vi "Launcher.vi"() -> ()   [LabVIEW 2024]
uses:
  Support/Traversal Type.ctl
  Tree_class/Tree.lvclass
  Iterator_interface/Iterator.lvclass
  <vilib>/Utility/miscctls.llb/LVRectTypeDef.ctl
  Node_class/Node.lvclass
panel:
  out "TreeSaved":bool
  in  "GoNext":bool
  in  "Save":bool
  in  "Add":bool
  in  "Value":dbl
  in  "TraversalType":T1
  out "TreeElements":dbl[](array[numeric])
  # "TREE VALUES"
  # "Made by Ramazan Burak Korkmaz"
  # "Value"
  # "Traversal\nType"
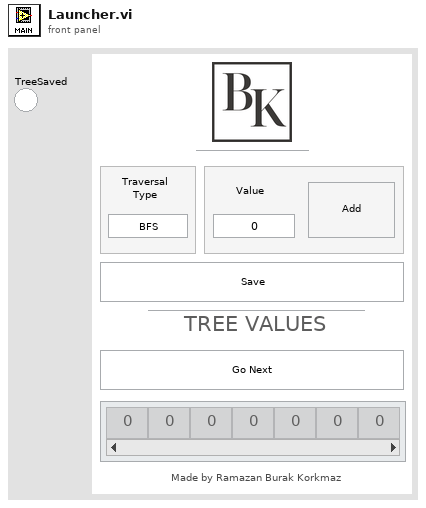
[diagram p1: front panel]
types:
  T1 = typedef "Traversal Type.ctl" = enum16{"BFS", "DFS"}
  T2 = enum8{"Enabled", "Disabled", "Disabled and Grayed Out"}
  T3 = typedef "LVRectTypeDef.ctl" = cluster{"Left":i16, "Top":i16, "Right":i16, "Bottom":i16}
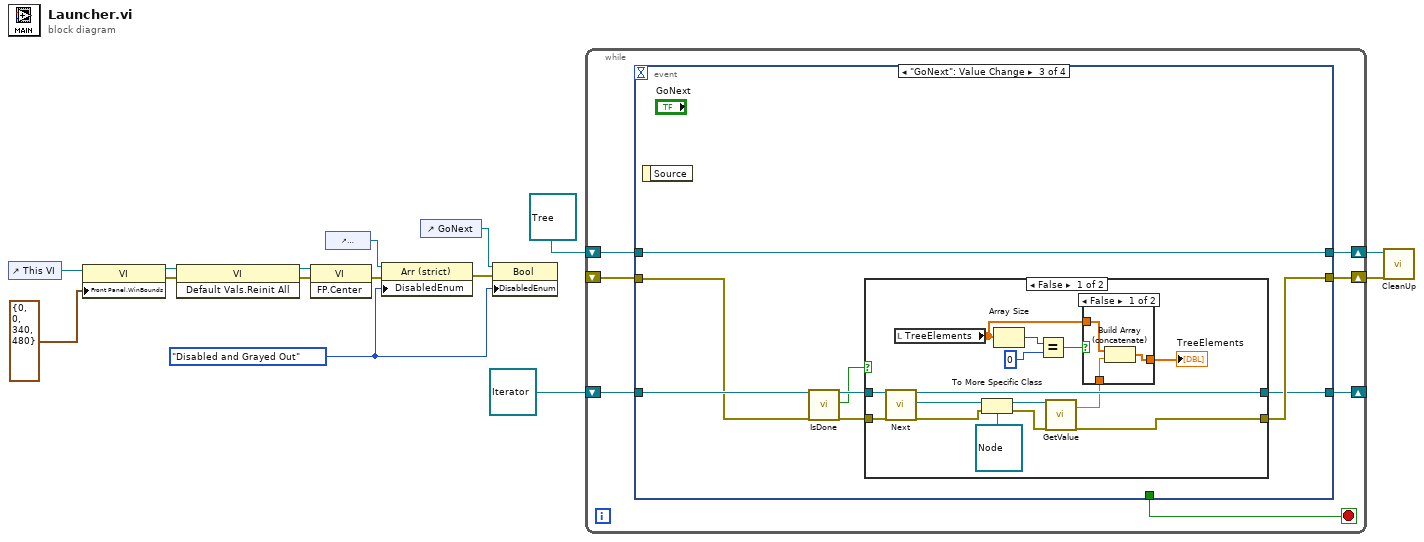
[diagram p0: block diagram]
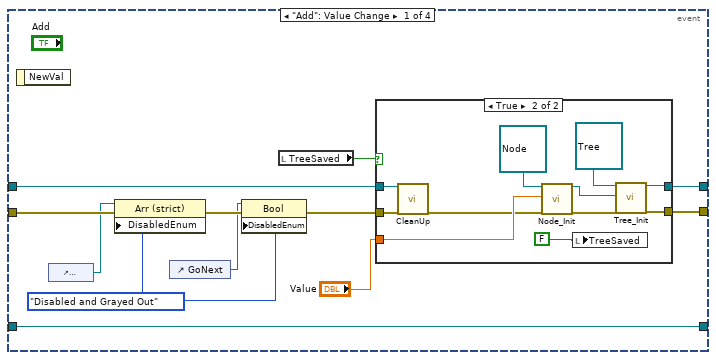
[diagram p2: hidden frame]
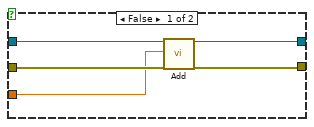
[diagram p3: hidden frame]
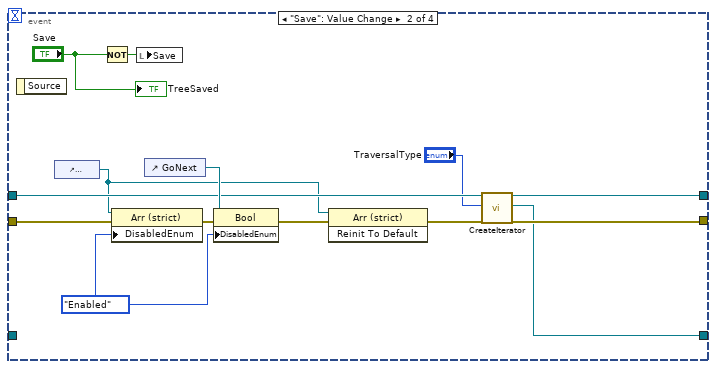
[diagram p4: hidden frame]
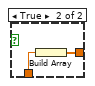
[diagram p5: hidden frame]
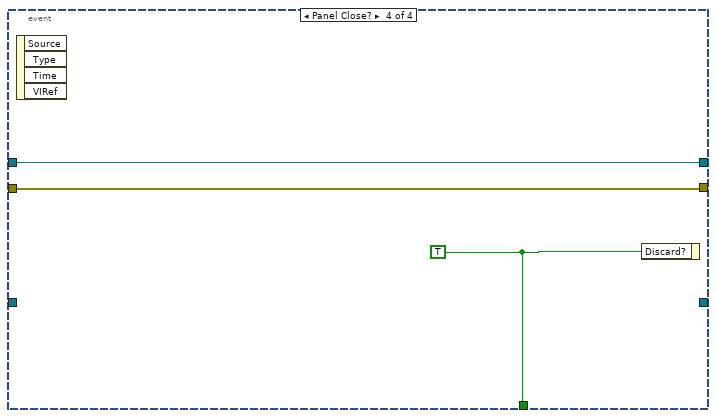
[diagram p7: hidden frame]
diagram:
  w7 = T2."Disabled and Grayed Out" ("Disabled")
  n1 = control-ref of="This VI"() -> (w13:refnum<vi>)
  n2 = property class="VI"(reference=w13, "Front Panel.WinBounds"=T3 {"Left"=0, "Top"=0, "Right"=340, "Bottom"=480} ("Front Panel Window:Window Bounds")) -> (reference out=w11:refnum<vi>, error out=w10:errorcluster)  [unwired: 1 in]
  n3 = invoke class="VI" method="Default Vals.Reinit All"(reference=w11, error in=w10) -> (reference out=w9:refnum<vi>, error out=w8:errorcluster)  [unwired: 1 in, 1 out]
  n4 = invoke class="VI" method="FP.Center"(reference=w9, error in=w8) -> (error out=w4:errorcluster)  [unwired: 1 in, 2 out]
  n5 = control-ref of="TreeElements"() -> (w5:refnum<vi>)
  n6 = property class="Arr (strict)"(reference=w5, error in=w4, "DisabledEnum"=w7) -> (error out=w3:errorcluster)  [unwired: 1 out]
  n7 = control-ref of="GoNext"() -> (w6:refnum<vi>)
  n8 = property class="Bool"(reference=w6, error in=w3, "DisabledEnum"=w7) -> ()  [unwired: 2 out]
  n9 = while {
    shift-right: [w20] -> w2
    shift-left: refnum<class "Tree.lvclass"> refnum ("Tree") -> [w22]
    shift-right: [w19] -> w1
    shift-left: _ -> [w21]
    shift-right: [w17] -> _
    shift-left: refnum<class "Iterator.lvclass"> refnum ("object out") -> [w16]
    stop <- w18 stop-if-true
    n10 = event shown="[2] \"GoNext\": Value Change" {
      selector: _ -> [_ _ _ _]
      dyn-events: _ -> [_ _ _ _]
      timeout: _ -> [_ _ _ _]
      tunnel: w22 -> [w31 w58 w69 w95]
      tunnel: w21 -> [w34 w64 w67 w97]
      tunnel: [w32 w57 w69 w95] -> w20
      tunnel: [w33 w59 w66 w97] -> w19
      tunnel: [_ _ _ w96] -> w18
      tunnel: [w23 w55 w65 _] -> w17
      tunnel: w16 -> [w23 _ w68 _]
      event "Add": Value Change {
        w25 = T2."Disabled and Grayed Out" ("Disabled")
        n11 = event-data() -> ()  [unwired: 1 in, 1 out]
        n12 = control-ref of="TreeElements"() -> (w28:refnum<vi>)
        n13 = property class="Arr (strict)"(reference=w28, error in=w34, "DisabledEnum"=w25) -> (error out=w29:errorcluster)  [unwired: 1 out]
        n14 = control-ref of="GoNext"() -> (w26:refnum<vi>)
        n15 = property class="Bool"(reference=w26, error in=w29, "DisabledEnum"=w25) -> (error out=w27:errorcluster)  [unwired: 1 out]
        n16 = local read "TreeSaved"() -> (w24:bool)
        n17 = case shown="True" w24 {
          tunnel: w27 -> [w39 w42]
          tunnel: [w38 w44] -> w33
          tunnel: [w37 w45] -> w32
          tunnel: w31 -> [w36 w43]
          tunnel: "Value" -> [w35 w50]
          frame False {
            n18 = call-dynamic "Add.vi"("object in"=w36, "Value"=w35, "Error In"=w39) -> ("object out"=w37:refnum<class "Tree.lvclass">, "Error Out"=w38:errorcluster)  [unwired: 15 in]
          }
          frame True {
            n19 = call-dynamic "CleanUp.vi"("object in"=w43, "Error In"=w42) -> ("Error Out"=w41:errorcluster)  [unwired: 16 in, 1 out]
            n20 = call "Node_Init.vi"("object in"=refnum<class "Node.lvclass"> refnum ("Node"), "Value"=w50, "Error In"=w41) -> ("object out"=w46:refnum<class "Node.lvclass">, "Error Out"=w47:errorcluster)  [unwired: 15 in]
            n21 = local write "TreeSaved"(FALSE ("TreeSaved")) -> ()
            n22 = call "Tree_Init.vi"("object in"=refnum<class "Tree.lvclass"> refnum ("Tree"), "Root"=w46, "Error In"=w47) -> ("object out"=w45:refnum<class "Tree.lvclass">, "Error Out"=w44:errorcluster)  [unwired: 15 in]
          }
        }
      }
      event "Save": Value Change {
        w60 = T2."Enabled" ("Disabled")
        n23 = event-data() -> ()  [unwired: 1 in, 1 out]
        n24 = control-ref of="TreeElements"() -> (w53:refnum<vi>)
        n25 = Not(x="Save") -> (.not. x?=w51:bool)
        n26 = property class="Arr (strict)"(reference=w53, error in=w64, "DisabledEnum"=w60) -> (error out=w63:errorcluster)  [unwired: 1 out]
        n27 = local write "Save"(w51) -> ()
        n28 = control-ref of="GoNext"() -> (w61:refnum<vi>)
        n29 = property class="Bool"(reference=w61, error in=w63, "DisabledEnum"=w60) -> (error out=w62:errorcluster)  [unwired: 1 out]
        n30 = invoke class="Arr (strict)" method="Reinit To Default"(reference=w53, error in=w62) -> (error out=w54:errorcluster)  [unwired: 1 in, 2 out]
        n31 = call-dynamic "CreateIterator.vi"("object in"=w58, "TraversalType"="TraversalType", "Error In"=w54) -> ("object out"=w57:refnum<class "Tree.lvclass">, "Iterator"=w55:refnum<class "Iterator.lvclass">, "Error Out"=w59:errorcluster)  [unwired: 14 in]
        "TreeSaved" <- "Save"
      }
      event "GoNext": Value Change {
        n32 = event-data() -> ()  [unwired: 1 in, 1 out]
        n33 = call-dynamic "IsDone.vi"("object in"=w68, "Error In"=w67) -> ("object out"=w71:refnum<class "Iterator.lvclass">, "IsDone"=w70:bool, "Error Out"=w72:errorcluster)  [unwired: 15 in]
        n34 = case shown="False" w70 {
          tunnel: [w79 w93] -> w66
          tunnel: [w85 w94] -> w65
          tunnel: w72 -> [w83 w93]
          tunnel: w71 -> [w82 w94]
          frame False {
            n35 = call-dynamic "Next.vi"("object in"=w82, "Error In"=w83) -> ("object out"=w85:refnum<class "Iterator.lvclass">, "Next"=w84:refnum<class "Element.lvclass">, "Error Out"=w81:errorcluster)  [unwired: 15 in]
            n36 = local read "TreeElements"() -> (w73:dbl[])
            n37 = To More Specific Class(target class=refnum<class "Node.lvclass"> refnum ("Node"), reference=w84, error in=w81) -> (specific class reference=w87:refnum<class "Node.lvclass">, error out=w80:errorcluster)
            n38 = Array Size(array=w73) -> (size(s)=w76:i32)
            n39 = Equal?(x=w76, y=0) -> (x = y?=w74:bool)
            n40 = call-dynamic "GetValue.vi"("object in"=w87, "Error In"=w80) -> ("Value"=w77:dbl, "Error Out"=w79:errorcluster)  [unwired: 15 in, 1 out]
            n41 = case shown="False" w74 {
              tunnel: [w90 w92] -> w78
              tunnel: w77 -> [w89 w91]
              tunnel: w73 -> [w88 _]
              frame False {
                n42 = Build Array (concatenate)(w88, w89) -> (w90:dbl[])
              }
              frame True {
                n43 = Build Array(w91) -> (w92:dbl[])
              }
            }
            "TreeElements" <- w78
          }
          frame True {
          }
        }
      }
      event Panel Close? {
        w96 = TRUE ("Discard?")
        n44 = event-data() -> ()  [unwired: 1 in, 4 out]
        n45 = event-data("Discard?"=w96) -> ()  [unwired: 1 in, 1 out]
      }
    }
  }
  n46 = call-dynamic "CleanUp.vi"("object in"=w2, "Error In"=w1) -> ()  [unwired: 16 in, 2 out]
